vi "Create Connection Collection.vi"(5 "Connection.Collection":refnum<class "Connection.Collection.lvclass">, 8 "error in (no error)":errorcluster, 11 "Collection":refnum<class "Connection.lvclass">[](array[class])) -> (0 "error out":errorcluster, 3 "Connection.Collection":refnum<class "Connection.Collection.lvclass">)   [LabVIEW 2013, in "Connection_GOSPL.lvlib" / "Connection.Collection.lvclass"]
uses:
  Connection.Collection.lvclass
  Connection/Connection.lvclass
  incoming connection.ctl
  map.ctl
  Connection.Collection.lvclass/Connection.Collection.ctl
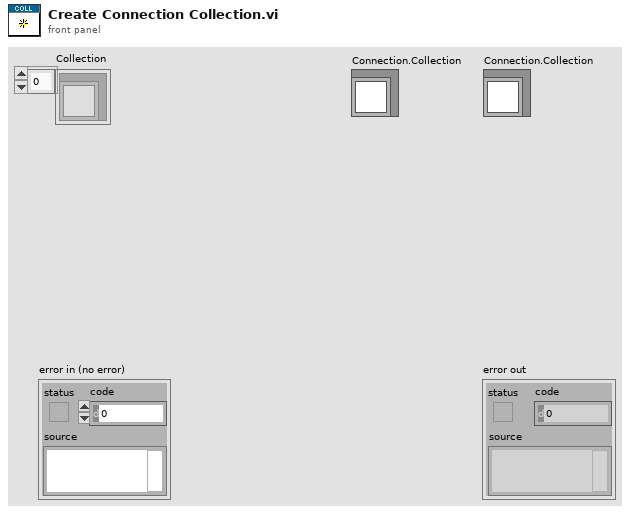
[diagram p1: front panel]
types:
  T1 = typedef "Connection_GOSPL.lvlib/Connection.Collection.lvclass/map.ctl" = cluster{"Connection":refnum<class "Connection.lvclass">, "Queue":refnum<queue>}
  T2 = typedef "Connection_GOSPL.lvlib/Connection.Collection.lvclass/incoming connection.ctl" = cluster{"Connection":refnum<class "Connection.lvclass">, "error":errorcluster}
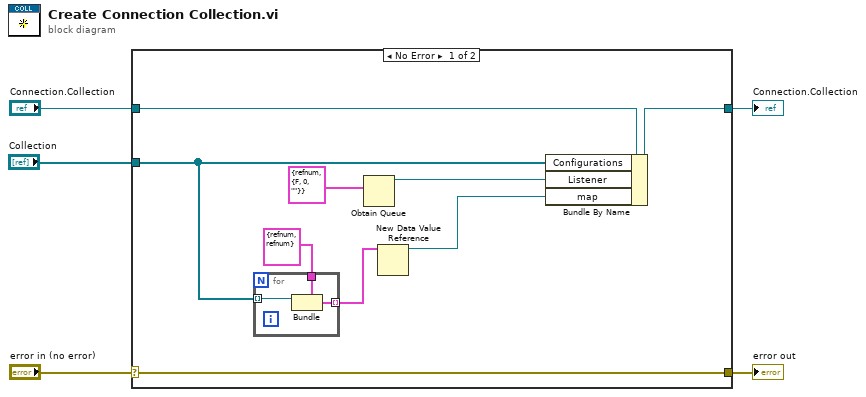
[diagram p0: block diagram]
diagram:
  n1 = case shown="No Error" "error in (no error)" {
    selector: "error in (no error)" -> [w13 w19]
    tunnel: [w13 w19] -> w4
    tunnel: [w12 w18] -> w2
    tunnel: "Connection.Collection" -> [w14 w18]
    tunnel: "Collection" -> [w8 _]
    frame No Error {
      n2 = for {
        tunnel: w8 -> [w17] mode=indexing
        tunnel: T1 {"Connection"=refnum, "Queue"=refnum} ("Map") -> [w16]
        tunnel: [w15] -> w6 mode=indexing
        n3 = Bundle(cluster=w16, "Connection"=w17) -> (w15:T1)  [unwired: 1 in]
      }
      n4 = Obtain Queue(element data type=T2 {"Connection"=refnum, "error"={"status"=FALSE, "code"=0, "source"=""}}) -> (queue out=w10:refnum<queue>)  [unwired: 4 in, 2 out]
      n5 = New Data Value Reference(data value=w6) -> (data value reference=w9:refnum<data-value>)  [unwired: 1 in, 1 out]
      n6 = Bundle By Name(cluster=w14, "Configurations"=w8, "Listener"=w10, "map"=w9) -> (w12:refnum<class "Connection.Collection.lvclass">)
    }
    frame Error {
    }
  }
  "error out" <- w4
  "Connection.Collection" <- w2
